vi "FT Write GPIO.vi"(0 "handle":u32, 5 "dir":u8, 7 "value":u8, 11 "error in (no error)":errorcluster) -> (4 "handle out":u32, 15 "error out":errorcluster)   [LabVIEW 2011, in "libMPSSE.lvlib"]
doc: "FTDI_API FT_STATUS FT_WriteGPIO(FT_HANDLE handle, uint8 dir, uint8 value);"
uses:
  libMPSSE.lvlib
  libMPSSE.dll
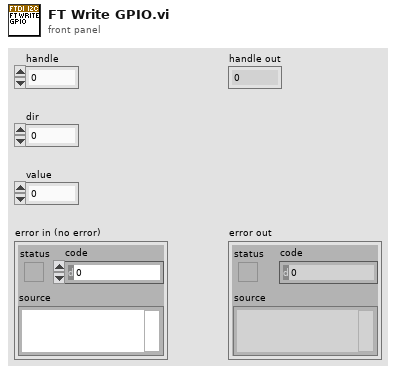
[diagram p1: front panel]
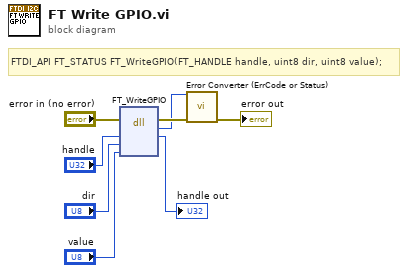
[diagram p0: block diagram]
diagram:
  # "FTDI_API FT_STATUS FT_WriteGPIO(FT_HANDLE handle, uint8 dir, uint8 value);"
  n1 = dll-call lib="D:/Project/HAL_Drivers/I2C/libMPSSE.*" fn="FT_WriteGPIO"(error in="error in (no error)", "handle"="handle", "dir"="dir", "value"="value") -> (error out=w3:errorcluster, w1:u32, "handle"=→"handle out":u32)  [unwired: 4 in, 1 out]
  n2 = call "Error Converter (ErrCode or Status).vi"("error code"=w1, "error in (no error)"=w3) -> ("error out"=→"error out":errorcluster)  [unwired: 13 in]
